vi "RemoveEctopicBeats.vi"(9 "X in [s]":dbl[](array[numeric]), 10 "RR intervals in [s]":dbl[](array[numeric])) -> (2 "RR intervals out [s]":dbl[](array[numeric]))   [LabVIEW 2014, in "Phonocardiography.lvlib"]
uses:
  Phonocardiography.lvlib
  <vilib>/gmath/NI_Gmath.lvlib
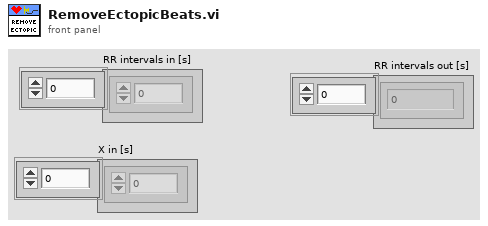
[diagram p1: front panel]
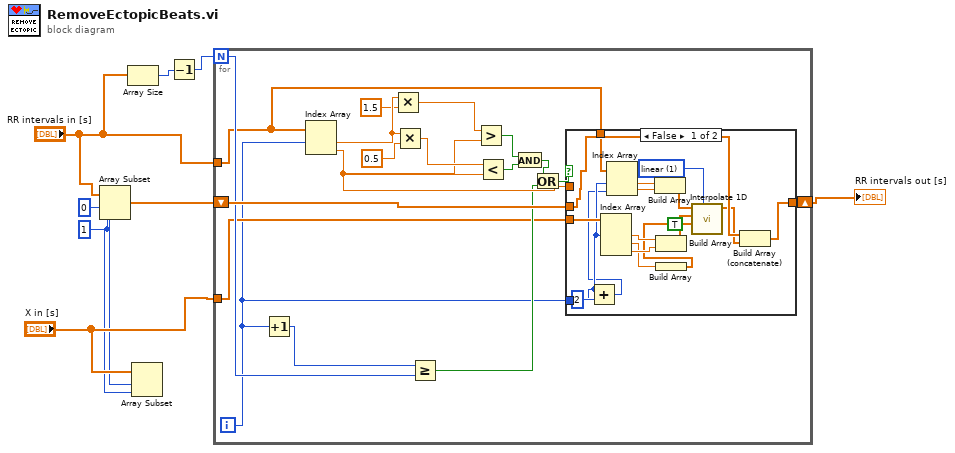
[diagram p0: block diagram]
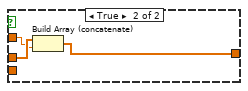
[diagram p2: hidden frame]
diagram:
  w1 = 1 ("length")
  w2 = 0 ("index")
  n1 = Array Subset(array="RR intervals in [s]", index=w2, length=w1) -> (w8:dbl[])
  n2 = Array Size(array="RR intervals in [s]") -> (size(s)=w5:i32)
  n3 = Array Subset(array="X in [s]", index=w2, length=w1) -> ()  [unwired: 1 out]
  n4 = Decrement(x=w5) -> (x-1=w4:i32)
  n5 = for {
    N: w4 -> [w17]
    tunnel: "RR intervals in [s]" -> [w9]
    shift-right: [w19] -> w7
    shift-left: w8 -> [w21]
    tunnel: "X in [s]" -> [w11]
    i -> [w10]
    n6 = Increment(x=w10) -> (x+1=w18:i32)
    n7 = Index Array(array=w9, index #1=w10) -> (element #1=w26:dbl, element #2=w20:dbl)  [unwired: 1 in]
    n8 = Multiply(x=w26, y=1.5) -> (x*y=w23:dbl)
    n9 = Multiply(x=w26, y=0.5) -> (x*y=w22:dbl)
    n10 = Greater Or Equal?(x=w18, y=w17) -> (x >= y?=w12:bool)
    n11 = Greater?(x=w23, y=w20) -> (0:w16:bool)
    n12 = Less?(x=w22, y=w20) -> (x < y?=w15:bool)
    n13 = And(x=w16, y=w15) -> (x .and. y?=w13:bool)
    n14 = Or(x=w13, y=w12) -> (x .or. y?=w14:bool)
    n15 = case shown="False" w14 {
      tunnel: w21 -> [w30 w47]
      tunnel: w20 -> [_ w46]
      tunnel: [w27 w45] -> w19
      tunnel: w11 -> [w44 _]
      tunnel: w10 -> [w42 _]
      tunnel: w9 -> [w29 _]
      frame False {
        w32 = 1 items=["nearest", "linear", "spline", "cubic Hermite", "Lagrange"] ("method")
        n16 = Add(x=w42, y=2) -> (x+y=w38:i32)
        n17 = Index Array(array=w44, index #1=w42) -> (element #1=w39:dbl, element #2=w36:dbl, element #3=w37:dbl)  [unwired: 2 in]
        n18 = Index Array(array=w29, index #1=w42, index #2=w38) -> (element #1=w41:dbl, element #2=w40:dbl)
        n19 = Build Array(w41, w40) -> (w33:dbl[])
        n20 = Build Array(w39, w37) -> (w34:dbl[])
        n21 = Build Array(w36) -> (w35:dbl[])
        n22 = call <vilib>:"Interpolate 1D.vi"("method"=w32, "X is monotonic"=TRUE, "xi"=w35, "X"=w34, "Y"=w33) -> ("yi"=w28:dbl[])  [unwired: 4 in, 2 out]
        n23 = Build Array (concatenate)(w30, w28) -> (w27:dbl[])
      }
      frame True {
        n24 = Build Array (concatenate)(w47, w46) -> (w45:dbl[])
      }
    }
  }
  "RR intervals out [s]" <- w7
